vi "DLPIO20 Write-Read-orig.vi"(5 "Write Buffer":u8[](array[numeric])=[2, 40] format="%x", 6 "Device Index":u32) -> (0 "Read Buffer Out":u8[](array[numeric]) format="%x", 3 "Bytes Read":u32, 4 "Bytes Written":u32=2)   [LabVIEW 2013]
uses:
  Global 1.vi
panel:
  out "Device Description":string="DLP-IO20"
  out "Bytes Waiting":u32
  # "Enter values in Write Buffer and run program.  \nWith a loop-back connector, the data is read back into the Read Buffer."
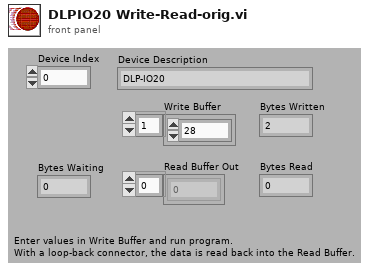
[diagram p1: front panel]
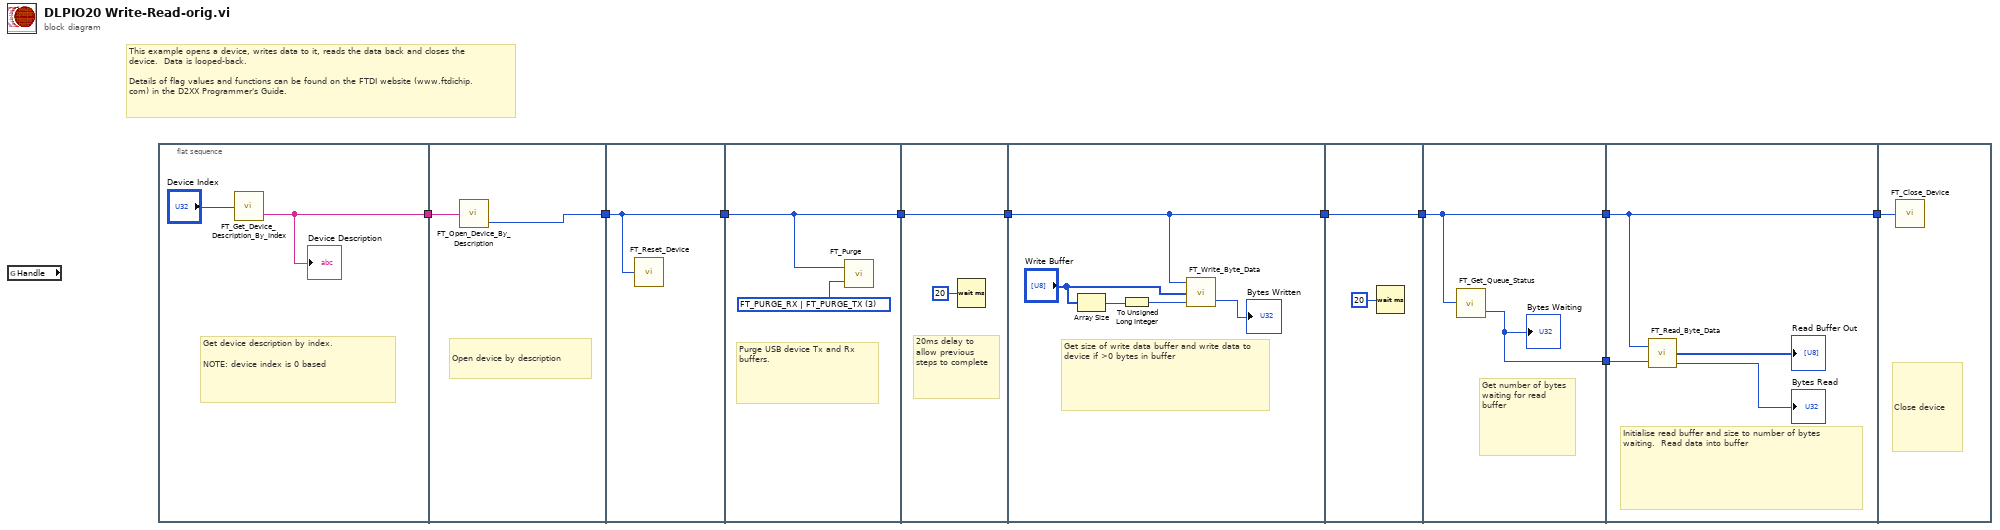
[diagram p0: block diagram]
diagram:
  # "This example opens a device, writes data to it, reads the data back and closes the device.  Data is looped-back.\n\nDetails of flag values and functions can be found on the FTDI website (www.ftdichip.com) in the D2XX Programmer's Guide."
  n1 = global read "Global 1.vi" "Handle"() -> ()  [unwired: 1 out]
  n2 = flat-sequence {
    tunnel: [w12] -> w7
    tunnel: [w14] -> w6
    tunnel: w7 -> [w13]
    tunnel: w6 -> [w15]
    tunnel: [w15] -> w2
    tunnel: [w16] -> w3
    tunnel: w2 -> [w16]
    tunnel: w3 -> [w18]
    tunnel: [w18] -> w1
    tunnel: [w20] -> w5
    tunnel: w1 -> [w20]
    tunnel: w5 -> [w26]
    tunnel: [w26] -> w10
    tunnel: w10 -> [w28]
    tunnel: [w28] -> w9
    tunnel: [w27] -> w8
    tunnel: w9 -> [w31]
    tunnel: [w31] -> w4
    tunnel: w8 -> [w29]
    tunnel: w4 -> [w33]
    frame #0 {
      # "Get device description by index.\n\nNOTE: device index is 0 based"
      n3 = call "FT_Get_Device_Description_By_Index.vi"("Device Index"="Device Index") -> ("Device Description"=w12:string)  [unwired: 1 out]
      "Device Description" <- w12
    }
    frame #1 {
      # "Open device by description"
      n4 = call "FT_Open_Device_By_Description.vi"("Device Description"=w13) -> ("Handle"=w14:u32)  [unwired: 1 out]
    }
    frame #2 {
      n5 = call "FT_Reset_Device.vi"("Handle"=w15) -> ()  [unwired: 1 out]
    }
    frame #3 {
      w17 = u32 3 items=["FT_PURGE_RX"=1, "FT_PURGE_TX"=2, "FT_PURGE_RX | FT_PURGE_TX"=3] ("Purge Flags")
      # "Purge USB device Tx and Rx  buffers."
      n6 = call "FT_Purge.vi"("Purge Flags"=w17, "Handle"=w16) -> ()  [unwired: 1 out]
    }
    frame #4 {
      # "20ms delay to allow previous steps to complete"
      n7 = Wait (ms)(milliseconds to wait=u32 20) -> ()  [unwired: 1 out]
    }
    frame #5 {
      # "Get size of write data buffer and write data to device if >0 bytes in buffer"
      n8 = Array Size(array="Write Buffer") -> (size(s)=w21:i32)
      n9 = To Unsigned Long Integer(number=w21) -> (unsigned 32bit integer=w22:u32)
      n10 = call "FT_Write_Byte_Data.vi"("Bytes To Write"=w22, "Buffer"="Write Buffer", "Handle"=w20) -> ("Bytes Written"=→"Bytes Written":u32)  [unwired: 1 out]
    }
    frame #6 {
      n11 = Wait (ms)(milliseconds to wait=u32 20) -> ()  [unwired: 1 out]
    }
    frame #7 {
      # "Get number of bytes waiting for read buffer"
      n12 = call "FT_Get_Queue_Status.vi"("Handle"=w28) -> ("Bytes Waiting"=w27:u32)  [unwired: 1 out]
      "Bytes Waiting" <- w27
    }
    frame #8 {
      # "Initialise read buffer and size to number of bytes waiting.  Read data into buffer"
      n13 = call "FT_Read_Byte_Data.vi"("Handle"=w31, "Bytes To Read"=w29) -> ("Read Data"=→"Read Buffer Out":u8[], "Bytes Read"=→"Bytes Read":u32)  [unwired: 1 out]
    }
    frame #9 {
      # "Close device"
      n14 = call "FT_Close_Device.vi"("Handle"=w33) -> ()  [unwired: 1 out]
    }
  }
